vi "PPT_get_rdg.vi"(4 "Channel Name":string, 7 "Address":T1) -> (1 "Reading":dbl format="%.3f", 3 "Comment":string)   [LabVIEW 2010]
uses:
  ADAM Client/Sub VIs/ADAM Controls/Address.ctl
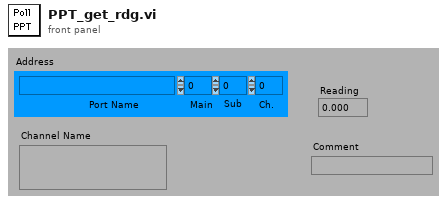
[diagram p1: front panel]
types:
  T1 = typedef "Address.ctl" = cluster{"Main":i32, "Ch.":i32, "Sub":i32, "Port Name":string}
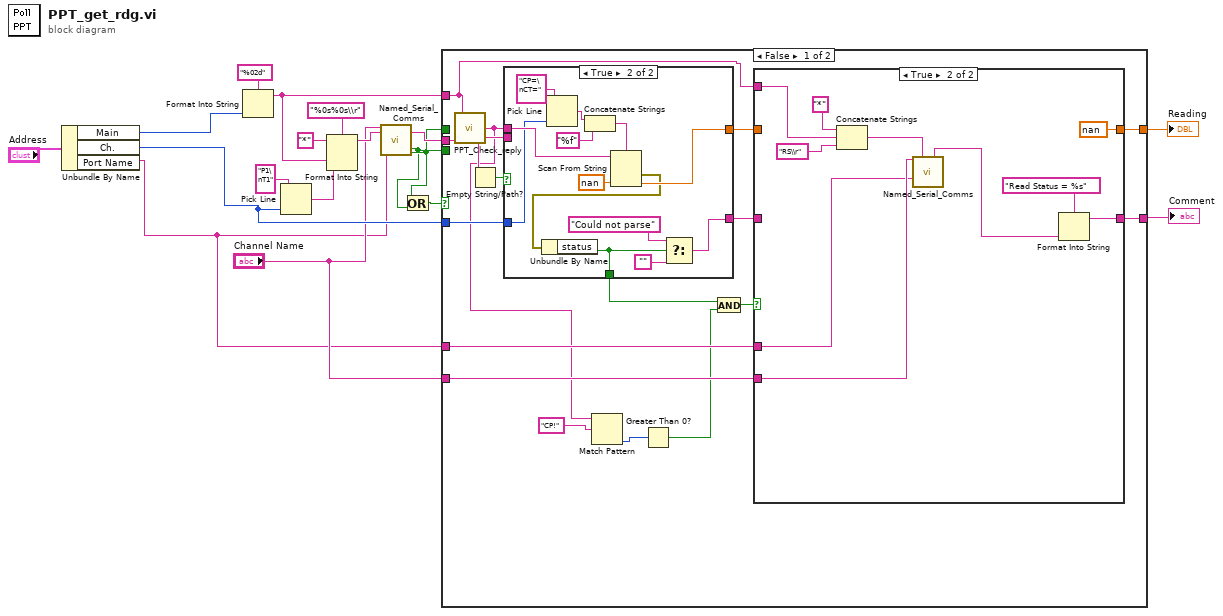
[diagram p0: block diagram]
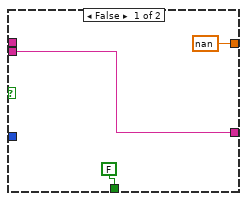
[diagram p3: hidden frame]
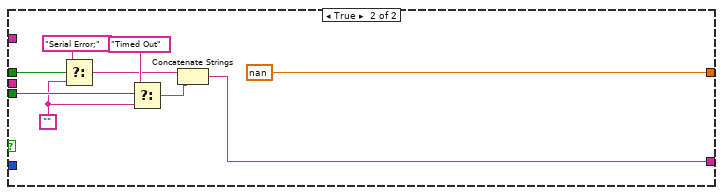
[diagram p4: hidden frame]
diagram:
  n1 = Unbundle By Name("Address") -> ("Main"=w4:i32, "Ch."=w3:i32, "Port Name"=w1:string)
  n2 = Format Into String(format string="%02d", w4) -> (resulting string=w8:string)  [unwired: 2 in, 1 out]
  n3 = Pick Line(multi-line string="P1\nT1", line index=w3) -> (output string=w15:string)  [unwired: 1 out]
  n4 = Format Into String(format string="%0s%0s\\r", initial string="*", w8, w15) -> (resulting string=w9:string)  [unwired: 1 in, 1 out]
  n5 = call "Named_Serial_Comms.vi"("Channel Name"="Channel Name", "Write String"=w9, "Port Name"=w1) -> ("Read"=w13:string, "Timed out"=w10:bool, "Serial Error"=w11:bool)  [unwired: 6 in, 4 out]
  n6 = Or(x=w11, y=w10) -> (x .or. y?=w12:bool)
  n7 = case shown="False" w12 {
    tunnel: [w29 w65] -> w6
    tunnel: w13 -> [w35 _]
    tunnel: [w30 nan] -> w7
    tunnel: w11 -> [_ w71]
    tunnel: w10 -> [_ w69]
    tunnel: w8 -> [w27 _]
    tunnel: w3 -> [w32 _]
    tunnel: "Channel Name" -> [w26 _]
    tunnel: w1 -> [w25 _]
    frame False {
      n8 = call "PPT_Check_reply.vi"("Address"=w27, "PPT reply"=w35) -> ("Stripped string"=w23:string, "Error Notes"=w33:string)  [unwired: 1 out]
      n9 = Empty String/Path?(string/path=w33) -> (empty?=w34:bool)
      n10 = case shown="True" w34 {
        tunnel: [nan w59] -> w31
        tunnel: w23 -> [_ w57]
        tunnel: [w50 w54] -> w28
        tunnel: w33 -> [w50 _]
        tunnel: w32 -> [_ w56]
        tunnel: [FALSE ("status") w51] -> w21
        frame False {
        }
        frame True {
          n11 = Pick Line(multi-line string="CP=\nCT=", line index=w56) -> (output string=w63:string)  [unwired: 1 out]
          n12 = Concatenate Strings(w63, "%f") -> (w58:string)
          n13 = Scan From String(format string=w58, input string=w57, default 1=nan ("Reading")) -> (error out=w55:errorcluster, output 1=w59:dbl)  [unwired: 2 in, 2 out]
          n14 = Unbundle By Name(w55) -> ("status"=w51:bool)
          n15 = Select(t="Could not parse", s=w51, f="") -> (s? t:f=w54:string)
        }
      }
      n16 = Match Pattern(string=w23, regular expression="CP!") -> (offset past match=w22:i32)  [unwired: 4 out]
      n17 = Greater Than 0?(x=w22) -> (x > 0?=w20:bool)
      n18 = And(x=w21, y=w20) -> (x .and. y?=w19:bool)
      n19 = case shown="True" w19 {
        tunnel: w31 -> [w37 _]
        tunnel: [w37 nan ("Reading")] -> w30
        tunnel: [w36 w38] -> w29
        tunnel: w28 -> [w36 _]
        tunnel: w27 -> [_ w46]
        tunnel: w26 -> [_ w44]
        tunnel: w25 -> [_ w42]
        frame False {
        }
        frame True {
          n20 = Concatenate Strings("*", w46, "RS\\r" ("string")) -> (w43:string)
          n21 = call "Named_Serial_Comms.vi"("Channel Name"=w44, "Write String"=w43, "Port Name"=w42) -> ("Read"=w40:string)  [unwired: 6 in, 6 out]
          n22 = Format Into String(format string="Read Status = %s", w40) -> (resulting string=w38:string)  [unwired: 2 in, 1 out]
        }
      }
    }
    frame True {
      w64 = ""
      n23 = Select(t="Serial Error;", s=w71, f=w64) -> (s? t:f=w67:string)
      n24 = Select(t="Timed Out", s=w69, f=w64) -> (s? t:f=w66:string)
      n25 = Concatenate Strings(w67, w66) -> (w65:string)
    }
  }
  "Reading" <- w7
  "Comment" <- w6
